vi "libdaq_adc_clear_buffer.vi"(0 "error in (no error)":errorcluster, 1 "device_name":string, 2 "module_name":string) -> (14 "error out":errorcluster, 15 "device_name":string, 16 "module_name":string)   [LabVIEW 2010, in "libdaqVI.lvlib"]
doc: "清除ADC模块的缓冲区数据，包括硬件缓冲区和软件缓冲区，在开启一个新的采样任务之前建议进行一次清空缓冲区的操作，避免前一次未读取完的数据误认为是本次采样数据，影响采样结果"
uses:
  libdaqVI.lvlib
  dll/daqlib.dll
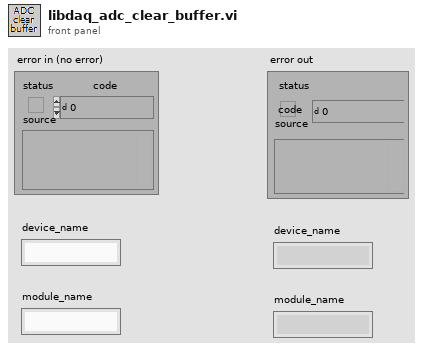
[diagram p1: front panel]
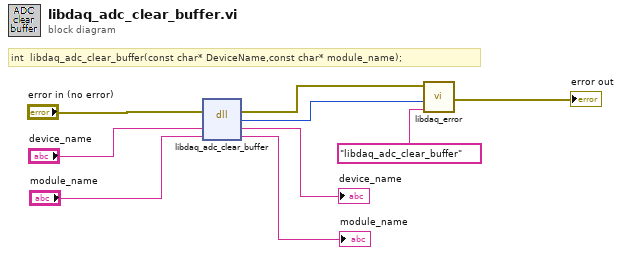
[diagram p0: block diagram]
diagram:
  # "int  libdaq_adc_clear_buffer(const char* DeviceName,const char* module_name);"
  n1 = dll-call lib="E:/Product/Example/DAQ-USB3212/Labview/labview_2010/libdaqVI/dll/daqlib.dll" fn="libdaq_adc_clear_buffer"(error in="error in (no error)", "device_name"="device_name", "module_name"="module_name") -> (error out=w4:errorcluster, "return type"=w3:i32, "device_name"=→"device_name":string, "module_name"=→"module_name":string)  [unwired: 2 in, 1 out]
  n2 = call "libdaq_error.vi"("error source"="libdaq_adc_clear_buffer", "error code"=w3, "错误输入（无错误）"=w4) -> ("错误输出"=→"error out":errorcluster)  [unwired: 8 in]
